vi "add_CRC.vi"(1 "Raw Data":u8[](array[numeric])) -> (0 "Data + CRC":u8[](array[numeric]))   [LabVIEW 2022 SP3]
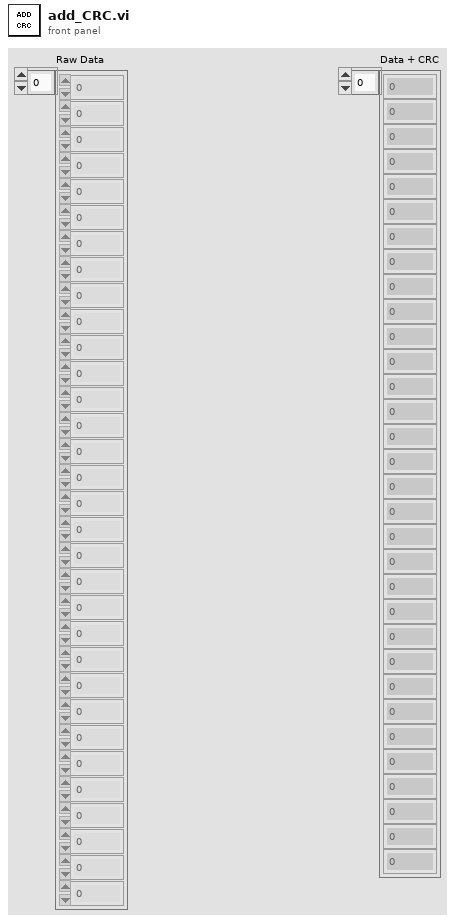
[diagram p1: front panel]
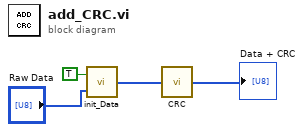
[diagram p0: block diagram]
diagram:
  n1 = call "init_Data.vi"("Input"="Raw Data", "Zerar CRC"=TRUE) -> ("Output"=w2:u8[])
  n2 = call "CRC.vi"("Data"=w2) -> ("Data + CRC"=→"Data + CRC":u8[])
